vi "ImgDataQueueFGV.vi"(8 "error out":errorcluster, 9 "Data In":cluster{u16[], i32, i64}, 10 "timeout in ms (-1)":i32=-1, 11 "Action":T1(ring)=enum."Lossy Enqueue") -> (0 "error out 2":errorcluster, 1 "Data Out":cluster{u16[], i32, i64}, 2 "timed out?":bool=TRUE)   [LabVIEW 2015]
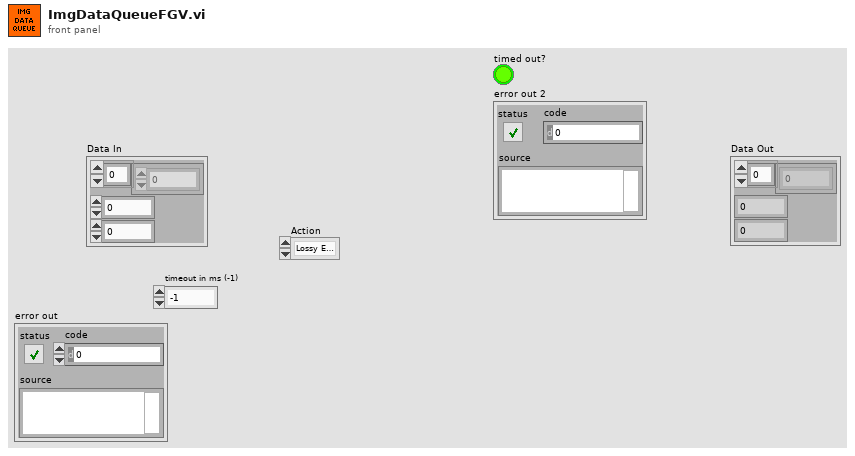
[diagram p1: front panel]
types:
  T1 = enum16{"Create", "Lossy Enqueue", "Enqueue", "Dequeue", "Destroy"}
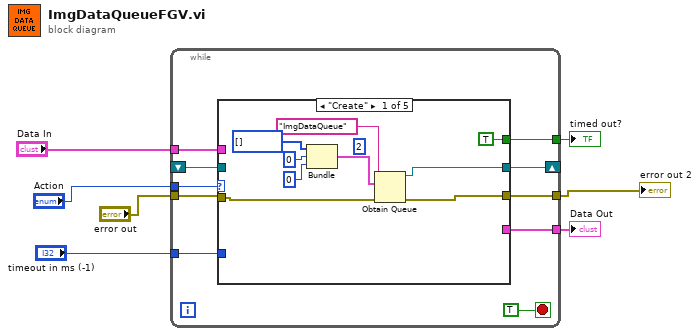
[diagram p0: block diagram]
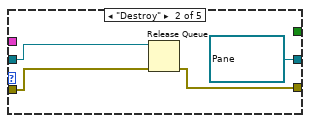
[diagram p2: hidden frame]
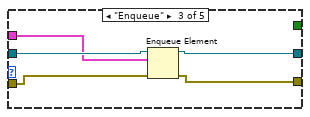
[diagram p3: hidden frame]
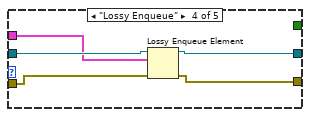
[diagram p4: hidden frame]
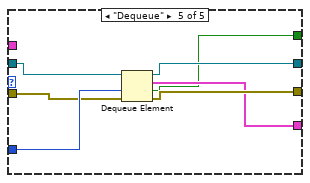
[diagram p5: hidden frame]
diagram:
  n1 = while {
    tunnel: "Action" -> [w17]
    shift-right: [w14] -> _
    shift-left: _ -> [w13]
    tunnel: "Data In" -> [w12]
    tunnel: "timeout in ms (-1)" -> [w11]
    tunnel: [w9] -> w4
    tunnel: [w8] -> w3
    tunnel: "error out" -> [w15]
    tunnel: [w16] -> w1
    stop <- TRUE stop-if-true
    n2 = case shown="\"Create\"" w17 {
      tunnel: [w26 w28 w32 w37 w45] -> w16
      tunnel: w15 -> [w25 w29 w33 w38 w44]
      tunnel: [w19 refnum<queue> refnum ("queue out") w34 w39 w43] -> w14
      tunnel: w13 -> [_ w30 w35 w40 w47]
      tunnel: w12 -> [_ _ w31 w36 _]
      tunnel: w11 -> [_ _ _ _ w46]
      tunnel: [_ _ _ _ w42] -> w9
      tunnel: [TRUE ("timed out?") _ _ _ w41] -> w8
      frame "Create" {
        (unwired) 2 ("max queue size (-1, unlimited)")
        n3 = Bundle(u16[] [], 0, i64 0) -> (w22:cluster{u16[], i32, i64})  [unwired: 1 in]
        n4 = Obtain Queue(name (unnamed)="ImgDataQueue", element data type=w22, error in (no error)=w25) -> (queue out=w19:refnum<queue>, error out=w26:errorcluster)  [unwired: 2 in, 1 out]
      }
      frame "Destroy" {
        n5 = Release Queue(queue=w30, error in (no error)=w29) -> (error out=w28:errorcluster)  [unwired: 1 in, 2 out]
      }
      frame "Enqueue" {
        n6 = Enqueue Element(queue=w35, element=w31, error in (no error)=w33) -> (queue out=w34:refnum<queue>, error out=w32:errorcluster)  [unwired: 1 in, 1 out]
      }
      frame "Lossy Enqueue" {
        n7 = Lossy Enqueue Element(queue=w40, element=w36, error in (no error)=w38) -> (queue out=w39:refnum<queue>, error out=w37:errorcluster)  [unwired: 2 out]
      }
      frame "Dequeue" {
        n8 = Dequeue Element(queue=w47, timeout in ms (-1)=w46, error in (no error)=w44) -> (queue out=w43:refnum<queue>, element=w42:cluster{u16[], i32, i64}, timed out?=w41:bool, error out=w45:errorcluster)
      }
    }
  }
  "Data Out" <- w4
  "timed out?" <- w3
  "error out 2" <- w1
